vi "MACBIN Verify Header__ogtk.vi"(8 "error in (no error)":errorcluster, 10 "macbinary file":path, 11 "data file":path) -> (0 "error out":errorcluster, 1 "file offset":i32, 2 "data file out":path, 3 "file refnum":refnum<file>, 4 "header bytes":u8[](array[numeric]), 5 "macbinary version":i32, 6 "macbinary header":T1 {"last mod" format="%<%I:%M:%S %p\n%d/%m/%y>T"; "creation date" format="%<%H:%M:%S\n%d/%m/%y>T"})   [LabVIEW 2011]
uses:
  MACBIN Macbinary Header__ogtk.ctl
  file/file.llb/Valid Path - Traditional__ogtk.vi
panel:
  in  "dummy header":T1 {"last mod" format="%<%I:%M:%S %p\n%d/%m/%y>T"; "creation date" format="%<%H:%M:%S\n%d/%m/%y>T"}
  # "Please visit http://www.OpenG.org to learn about the\nOpen Source LabVIEW software movement.\n\nNOTICE -- YOU MUST LEAVE THIS NOTICE IN PLACE.  PER THE TERMS OF THE LICENSE BELOW, YOU MAY SUBLICENSE THIS SOFTWARE \nIN ANY WAY THAT DOES NOT CONFLICT WITH THIS LICENSE.\n\n### BSD License (http://www.opensource.org/licenses/bsd-license.php) Begin ###\n \nCopyright (C) 2002 Christophe Salzmann christophe.salzmann@epfl.ch\nCopyright (C) 2002 Rolf Kalbermatter rolf.kalbermatter@citengineering.com\n\nAll rights reserved.\n\nRedistribution and use in source and binary forms, with or without modification, are permitted provided that the following conditions are met:\n\n    * Redistributions of source code must retain the above copyright notice, this list of conditions and the following disclaimer.\n    * Redistributions in binary form must reproduce the above copyright notice, this list of conditions and the following disclaimer in the \n       documentation and/or other materials provided with the distribution.\n    * Neither the name of SciWare, James Kring, Inc., nor the names of its contributors may be used to endorse or promote products derived \n       from this software without specific prior written permission.\n\nTHIS SOFTWARE IS PROVIDED BY THE COPYRIGHT HOLDERS AND CONTRIBUTORS \"AS IS\" AND ANY EXPRESS OR IMPLIED WARRANTIES, \nINCLUDING, BUT NOT LIMITED TO, THE IMPLIED WARRANTIES OF MERCHANTABILITY AND FITNESS FOR A PARTICULAR PURPOSE ARE \nDISCLAIMED. IN NO EVENT SHALL THE COPYRIGHT OWNER OR CONTRIBUTORS BE LIABLE FOR ANY DIRECT, INDIRECT, INCIDENTAL,\n SPECIAL, EXEMPLARY, OR CONSEQUENTIAL DAMAGES (INCLUDING, BUT NOT LIMITED TO, PROCUREMENT OF SUBSTITUTE GOODS OR \nSERVICES; LOSS OF USE, DATA, OR PROFITS; OR BUSINESS INTERRUPTION) HOWEVER CAUSED AND ON ANY THEORY OF LIABILITY, \nWHETHER IN CONTRACT, STRICT LIABILITY, OR TORT (INCLUDING NEGLIGENCE OR OTHERWISE) ARISING IN ANY WAY OUT OF THE USE \nOF THIS SOFTWARE, EVEN IF ADVISED OF THE POSSIBILITY OF SUCH DAMAGE.\n\n### BSD License End ###"
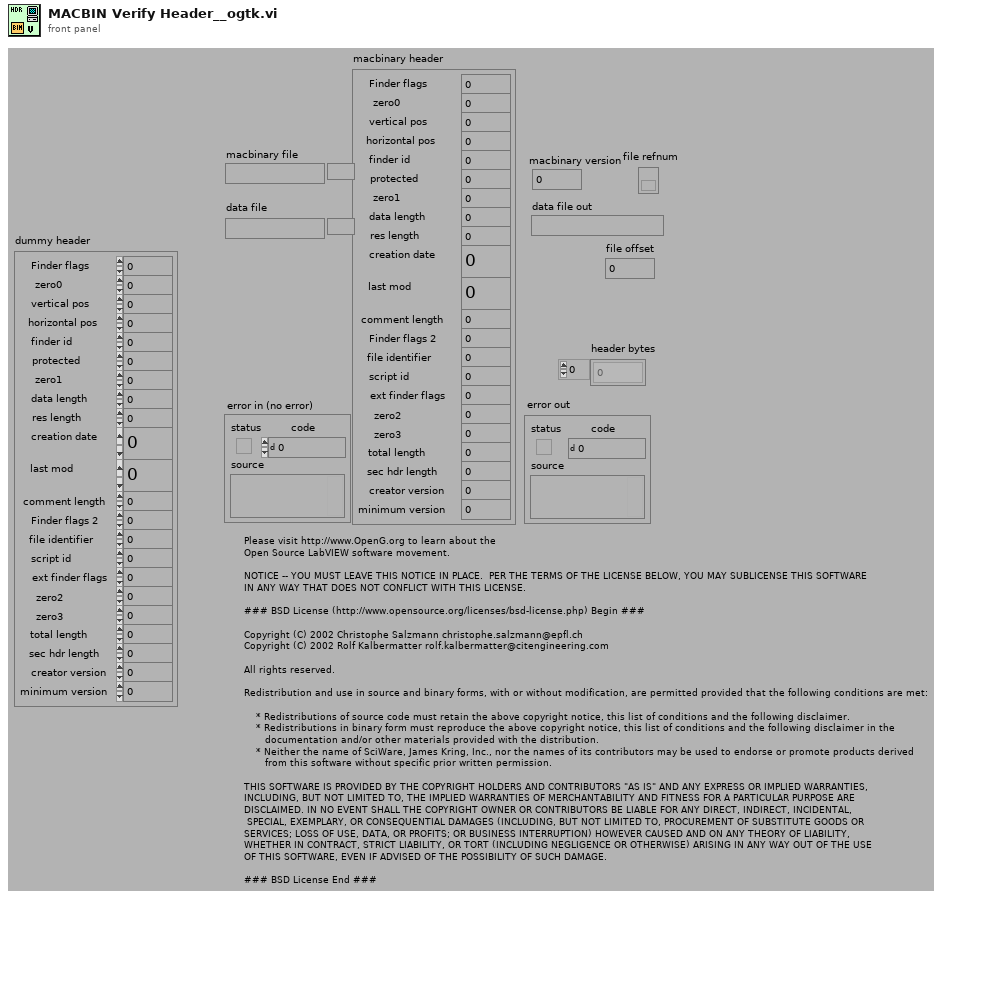
[diagram p1: front panel]
types:
  T1 = typedef "MACBIN Macbinary Header__ogtk.ctl" = cluster{"Finder flags":u8, "zero0":u8, "vertical pos":u16, "horizontal pos":u16, "finder id":u16, "protected":u8, "zero1":u8, "data length":i32, "res length":i32, "creation date":u32, "last mod":u32, "comment length":i16, "Finder flags 2":u8, "file identifier":u32, "script id":u8, "ext finder flags":u8, "zero2":i32, "zero3":i32, "total length":u32, "sec hdr length":u16, "creator version":u8, "minimum version":u8}
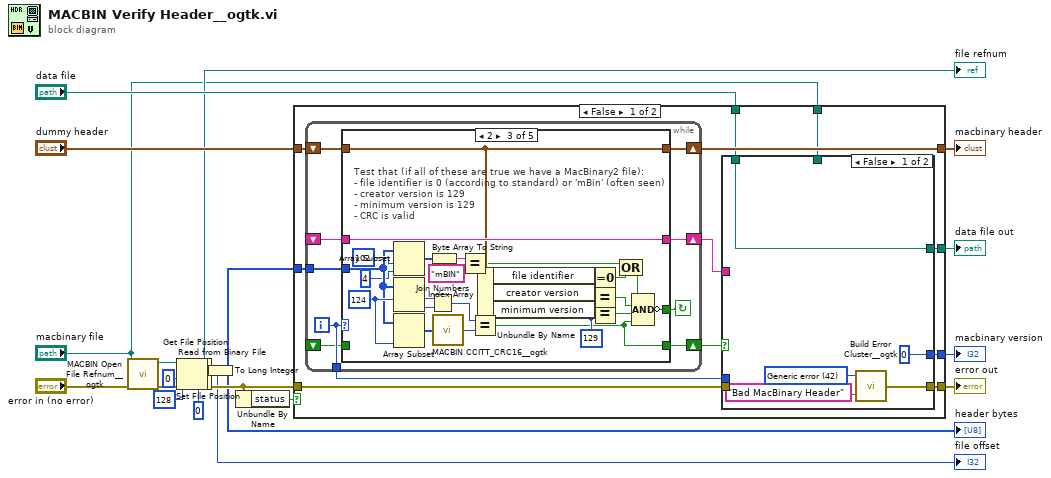
[diagram p0: block diagram]
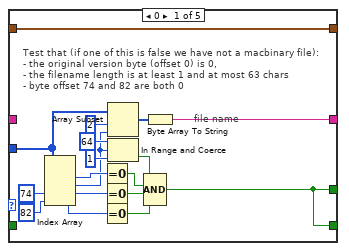
[diagram p2: hidden frame]
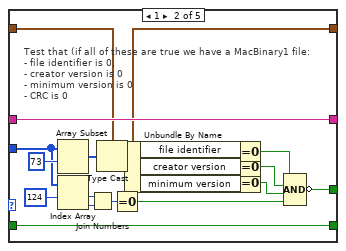
[diagram p3: hidden frame]
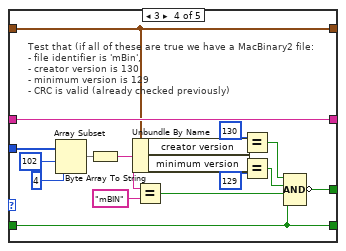
[diagram p4: hidden frame]
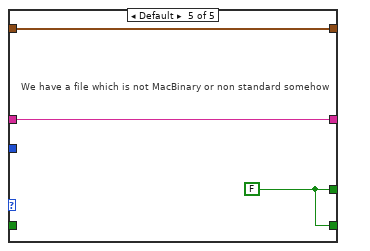
[diagram p5: hidden frame]
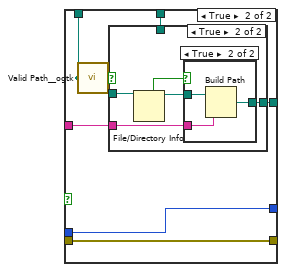
[diagram p6: hidden frame]
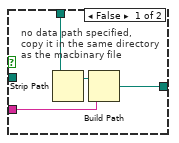
[diagram p7: hidden frame]
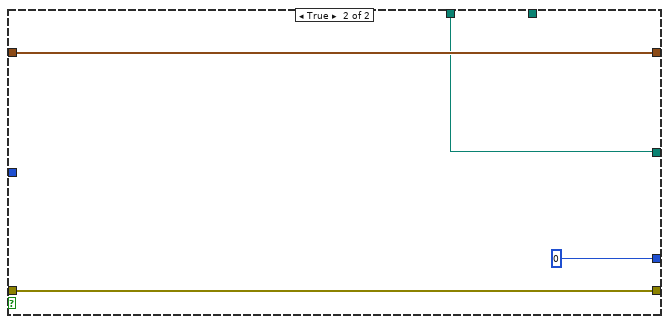
[diagram p9: hidden frame]
diagram:
  n1 = call "MACBIN Open File Refnum__ogtk.vi"("error in (no error)"="error in (no error)", "file path"="macbinary file") -> ("error out"=w16:errorcluster, "file refnum"=w17:refnum<file>)  [unwired: 5 in]
  n2 = Set File Position(offset (in bytes) (0)=0 ("pos offset (0)"), refnum=w17, error in=w16) -> (refnum out=w5:refnum<file>, error out=w4:errorcluster)  [unwired: 1 in]
  n3 = Read from Binary File(5:u8 0 ("Numeric"), 8:w4, 10:128 ("count"), 11:w5) -> (0:w2:errorcluster, 2:w9:u8[], 3:w3:refnum<file>)  [unwired: 2 in, 1 out]
  "header bytes" <- w9
  n4 = Get File Position(4:w2, 7:w3) -> (0:w12:errorcluster, 2:w1:i64, 3:→"file refnum":refnum<file>)
  n5 = To Long Integer(number=w1) -> (32bit integer=→"file offset":i32)
  n6 = Unbundle By Name(w12) -> ("status"=w20:bool)
  n7 = case shown="False" w20 {
    tunnel: [w35 0] -> w23
    tunnel: w9 -> [w32 _]
    tunnel: [w31 w155] -> w22
    tunnel: "dummy header" -> [w30 w155]
    tunnel: w12 -> [w28 w153]
    tunnel: [w27 w153] -> w19
    tunnel: "data file" -> [w26 w152]
    tunnel: [w25 w152] -> w6
    tunnel: "macbinary file" -> [w24 _]
    frame False {
      n8 = while {
        shift-left: _ -> [w37]
        shift-right: [w36] -> w29
        shift-left: w30 -> [w39]
        shift-right: [w38] -> w31
        shift-left: _ -> [w40]
        shift-right: [w41] -> w33
        tunnel: [w42] -> w34
        tunnel: w32 -> [w44]
        i -> [w42]
        stop <- w43 continue-if-true
        n9 = case shown="2" w42 {
          tunnel: w44 -> [w48 w78 w88 w117 _]
          tunnel: [w45 w67 w102 w122 w124] -> w43
          tunnel: [w47 w80 w106 w123 w126] -> w41
          tunnel: w40 -> [_ w80 w106 w123 w126]
          tunnel: w39 -> [w46 w64 w101 w121 w125]
          tunnel: [w46 w73 w101 w121 w125] -> w38
          tunnel: w37 -> [_ w63 _ w107 _]
          tunnel: [w45 w63 w91 w107 w124] -> w36
          frame 0 {
            # "Test that (if one of this is false we have not a macbinary file):\n- the original version byte (offset 0) is 0,\n- the filename length is at least 1 and at most 63 chars\n- byte offset 74 and 82 are both 0"
            # "file name"
            n10 = Index Array(array=w48, index #3=74 ("Index"), index #4=82 ("Index")) -> (element #1=w61:u8, element #2=w49:u8, element #3=w60:u8, element #4=w58:u8)  [unwired: 2 in]
            n11 = Equal To 0?(x=w61) -> (x = 0?=w56:bool)
            n12 = Equal To 0?(x=w60) -> (x = 0?=w57:bool)
            n13 = Equal To 0?(x=w58) -> (x = 0?=w55:bool)
            n14 = Array Subset(array=w48, index=2 ("Array Index"), length=w49) -> (w51:u8[])
            n15 = In Range and Coerce(upper limit=u8 64 ("y"), x=w49, lower limit=u8 1) -> (In Range?=w53:bool)  [unwired: 1 out]
            n16 = Compound Arithmetic op=AND(w53, w56, w57, w55) -> (w45:bool)
            n17 = Byte Array To String(unsigned byte array=w51) -> (string=w47:string)
          }
          frame 1 {
            # "Test that (if all of these are true we have a MacBinary1 file:\n- file identifier is 0,\n- creator version is 0\n- minimum version is 0\n- CRC is 0"
            n18 = Array Subset(array=w78, index=73 ("Array Index")) -> (w77:u8[])  [unwired: 1 in]
            n19 = Index Array(array=w78, index #1=124 ("Index")) -> (element #1=w75:u8, element #2=w76:u8)  [unwired: 1 in]
            n20 = Join Numbers(hi=w75, lo=w76) -> ((hi.lo)=w74:u16)
            n21 = Type Cast(type=w64, x=w77) -> (*(type *) &x=w73:T1)
            n22 = Equal To 0?(x=w74) -> (x = 0?=w65:bool)
            n23 = Unbundle By Name(w73) -> ("file identifier"=w72:u32, "creator version"=w70:u8, "minimum version"=w71:u8)
            n24 = Equal To 0?(x=w72) -> (x = 0?=w69:bool)
            n25 = Equal To 0?(x=w70) -> (x = 0?=w68:bool)
            n26 = Equal To 0?(x=w71) -> (x = 0?=w66:bool)
            n27 = Compound Arithmetic op=AND(w69, w68, w66, w65) -> (invert w67:bool)
          }
          frame 2 {
            w97 = u8 129 ("y")
            w94 = 124 ("Index")
            # "Test that (if all of these are true we have a MacBinary2 file):\n- file identifier is 0 (according to standard) or 'mBin' (often seen)\n- creator version is 129\n- minimum version is 129\n- CRC is valid"
            n28 = Array Subset(array=w88, index=102 ("Array Index"), length=4) -> (w89:u8[])
            n29 = Index Array(array=w88, index #1=w94) -> (element #1=w104:u8, element #2=w105:u8)  [unwired: 1 in]
            n30 = Array Subset(array=w88, length=w94) -> (w95:u8[])  [unwired: 1 in]
            n31 = Join Numbers(hi=w104, lo=w105) -> ((hi.lo)=w92:u16)
            n32 = Byte Array To String(unsigned byte array=w89) -> (string=w85:string)
            n33 = call "MACBIN CCITT_CRC16__ogtk.vi"("u8 array"=w95) -> ("Checksum"=w93:u16)  [unwired: 4 in]
            n34 = Equal?(x=w85, y="mBIN") -> (x = y?=w84:bool)
            n35 = Equal?(x=w92, y=w93) -> (x = y?=w91:bool)
            n36 = Unbundle By Name(w101) -> ("file identifier"=w103:u32, "creator version"=w100:u8, "minimum version"=w98:u8)
            n37 = Equal To 0?(x=w103) -> (x = 0?=w83:bool)
            n38 = Equal?(x=w100, y=w97) -> (x = y?=w99:bool)
            n39 = Equal?(x=w98, y=w97) -> (x = y?=w96:bool)
            n40 = Compound Arithmetic op=OR(w84, w83) -> (w82:bool)
            n41 = Compound Arithmetic op=AND(w82, w99, w96, w91) -> (invert w102:bool)
          }
          frame 3 {
            # "Test that (if all of these are true we have a MacBinary2 file:\n- file identifier is 'mBin',\n- creator version is 130\n- minimum version is 129\n- CRC is valid (already checked previously)"
            n42 = Array Subset(array=w117, index=102 ("Array Index"), length=4) -> (w109:u8[])
            n43 = Byte Array To String(unsigned byte array=w109) -> (string=w114:string)
            n44 = Unbundle By Name(w121) -> ("creator version"=w112:u8, "minimum version"=w120:u8)
            n45 = Equal?(x=w114, y="mBIN") -> (x = y?=w108:bool)
            n46 = Equal?(x=u8 130 ("y"), y=w112) -> (x = y?=w111:bool)
            n47 = Equal?(x=w120, y=u8 129) -> (x = y?=w110:bool)
            n48 = Compound Arithmetic op=AND(w111, w110, w108, w107) -> (invert w122:bool)
          }
          frame Default {
            w124 = FALSE
            # "We have a file which is not MacBinary or non standard somehow"
          }
        }
      }
      n49 = case shown="False" w29 {
        tunnel: [0 w138] -> w35
        tunnel: w34 -> [_ w138]
        tunnel: [w130 w137] -> w27
        tunnel: w28 -> [_ w137]
        tunnel: w26 -> [w127 w134]
        tunnel: w33 -> [_ w136]
        tunnel: [w127 w133] -> w25
        tunnel: w24 -> [_ w132]
        frame False {
          w129 = 42 items=["No error", "Argument error", "Memory is full", "Out of zone", "End of file", "File already open", "Generic file I/O error", "File not found", "File permission error", "Disk is full", "Duplicate path", "Too many files open", "System feature not enabled", "Resource file not found", "Cannot add resource", "Resource not found", "Image not found", "Image memory error", "Pen does not exist", "Config type invalid", "Config token not found", "Config parse error", "Config memory error", "Bad external code format", "Bad external code offset", "External code not present", "Null window", "Destroy window error", "Null menu", "Print aborted", "Bad print record", "Print driver error", "Windows error during printing", "Memory error during printing", "Print dialog error", "Generic print error", "Invalid device refnum", "Device not found", "Device parameter error", "Device unit error", "Cannot open device", "Device call aborted", "Generic error", "Cancelled by user", "Object ID too low", "Object ID too high", "Object not in heap", "Unknown heap", "Unknown object (invalid DefProc)", "Unknown object (DefProc not in table)", "Message out of range", "Invalid (null) method", "Unknown message", "Manager call not supported", "Bad address", "Network operation in progress", "Network operation timed out", "Connection is busy", "Network attribute not supported", "Network error", "Address in use", "System out of memory", "Connection aborted", "Connection refused", "Not connected", "Already connected", "Connection closed", "Initialization error (interapplication manager)", "Bad occurrence", "Wait on unbound occurrence handler", "Occurrence queue overflow", "Datalog type conflict", "Unused", "Unrecognized type (interapplication manager)", "Memory corrupt", "Failed to make temporary DLL", "Old CIN version", "Drag socket not found", "Failed to load drop-object", "Failed to register OLE object", "Failed to release OLE object", "Format specifier type mismatch", "Unknown format specifier", "Too few format specifiers", "Too many format specifiers", "Scan failed", "Newer CIN version", "Error converting to variant", "Runtime menu error", "Password tampered", "Variant attribute not found", "Incompatible variant data type", "Event data is not available", "Event Store is not present", "Occurrence is not found", "Event Queue is not created", "Event info is not available", "Refnum passed is NULL", "Error retrieving Class GUID", "Error retrieving CoClass GUID", "Error retrieving TypeLib GUID.", "Bad built application magic bytes.", "Specific driver is different from the specific driver associated with the Logical Name.", "There is no session opened to the class driver.", "Max Error", "MAX - Error with config objects", "MAX - Error loading configuration", "MAX - Group not supported"]
          n50 = call "Build Error Cluster__ogtk.vi"("String to Prepend to source (\"\")"="Bad MacBinary Header" ("String to Prepend to source (\"\")"), "code"=w129) -> ("error out"=w130:errorcluster)
        }
        frame True {
          n51 = call-poly "Valid Path__ogtk.vi"("path"=w134) -> ("valid"=w135:bool)
          n52 = case shown="True" w135 {
            tunnel: [w141 w144] -> w133
            tunnel: w136 -> [w140 w143]
            tunnel: w134 -> [_ w147]
            tunnel: w132 -> [w139 _]
            frame False {
              # "no data path specified,\ncopy it in the same directory\nas the macbinary file"
              n53 = Strip Path(path=w139) -> (stripped path=w142:path)  [unwired: 1 out]
              n54 = Build Path(base path=w142, name or relative path=w140) -> (appended path=w141:path)
            }
            frame True {
              n55 = File/Directory Info(path=w147) -> (path out=w145:path, directory=w146:bool)  [unwired: 1 in, 5 out]
              n56 = case shown="True" w146 {
                tunnel: w145 -> [w148 w149]
                tunnel: [w148 w151] -> w144
                tunnel: w143 -> [_ w150]
                frame False {
                }
                frame True {
                  n57 = Build Path(base path=w149, name or relative path=w150) -> (appended path=w151:path)
                }
              }
            }
          }
        }
      }
    }
    frame True {
    }
  }
  "macbinary version" <- w23
  "macbinary header" <- w22
  "error out" <- w19
  "data file out" <- w6
